vi "Stack1 Indicator.vi"() -> ()   [LabVIEW 2024]
uses:
  gitlab/imponator-series-actor/Imponator Series Actor/Imponator Series UI Actor/Progress Bar Switch.ctl
  gitlab/imponator-series-actor/Imponator Series Actor/Imponator Series UI Actor/Stack.ctl
panel:
  out "Stack1":T1 {"Power-Setpoint" format="%d %"; "Purge Valve" scale=0.0..100.0; "Supply Valve" scale=0.0..100.0; "Switch" scale=0.0..100.0; "Voltage" format="%#.2f V"; "Current" format="%#.2f A"; "Pressure" format="%#.0f mbar"; "Thermometer" format="%#.1f °C"; "Fan" format="%d %"; "Power" format="%d W"}
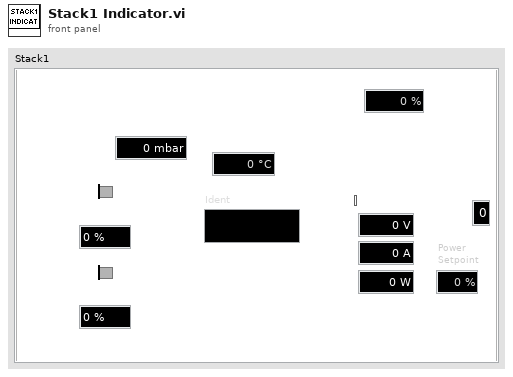
[diagram p1: front panel]
types:
  T1 = typedef "Stack.ctl" = cluster{"Ident":string, "Power":dbl, "Fan":dbl, "Thermometer":dbl, "MCU":u8, "Pressure":dbl, "Current":dbl, "Voltage":dbl, "Switch 2":bool, "Switch 3":bool, "Switch":T2, "Switch 4":bool, "Supply Valve":dbl, "Purge Valve":dbl, "Power-Setpoint":dbl}
  T2 = typedef "Progress Bar Switch.ctl" = u8
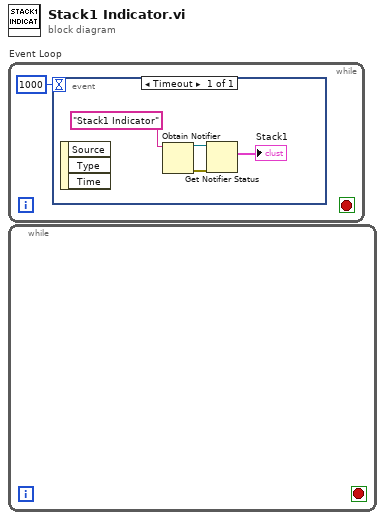
[diagram p0: block diagram]
diagram:
  n1 = while "Event Loop" {
    stop <- _ stop-if-true
    n2 = event shown="[0] Timeout" {
      selector: _ -> [_]
      dyn-events: _ -> [_]
      timeout: 1000 -> [_]
      event Timeout {
        n3 = event-data() -> ()  [unwired: 1 in, 3 out]
        n4 = Obtain Notifier(name (unnamed)="Stack1 Indicator") -> (notifier out=w3:refnum<notifier>, error out=w4:errorcluster)  [unwired: 3 in, 1 out]
        n5 = Get Notifier Status(notifier=w3, error in (no error)=w4) -> (current notification=→"Stack1":T1)  [unwired: 4 out]
      }
    }
  }
  n6 = while {
    stop <- _ stop-if-true
  }
